vi "WFDC Compute Z Calibration.vi"(0 "Scan Positions File Name":string="Scan Positions.xml", 1 "User Close?":bool=TRUE, 2 "Half Shift":i32=7, 7 "Data Path":path, 11 "Error":errorcluster) -> (4 "Fit Slope":dbl=0.02 format="%#_6f", 8 "Fit Intercept":dbl=0.02, 13 "Ref Images":T1[](array[typedef]), 15 "Error":errorcluster)   [LabVIEW 2020]
uses:
  <vilib>/vision/Image Controls.llb/IMAQ Image.ctl
  WFDC Controls/WFDC Reference Image Info.ctl
  <vilib>/Utility/miscctls.llb/LVPointTypeDef.ctl
  <vilib>/Analysis/6fits.llb/Curve Fitting Criteria.ctl
  WFDC DLL and Testing/Visual Studio NCC Max Shift DLL/x64/Release/VSmaxShiftNCC.dll
  <vilib>/Analysis/NI_AALPro.lvlib
panel:
  out "Z Calibration":cluster{dbl[], dbl[]}[](graph)
  in  "Done":bool
  out "Wait Bar":i32(slide) scale=0.0..11.0
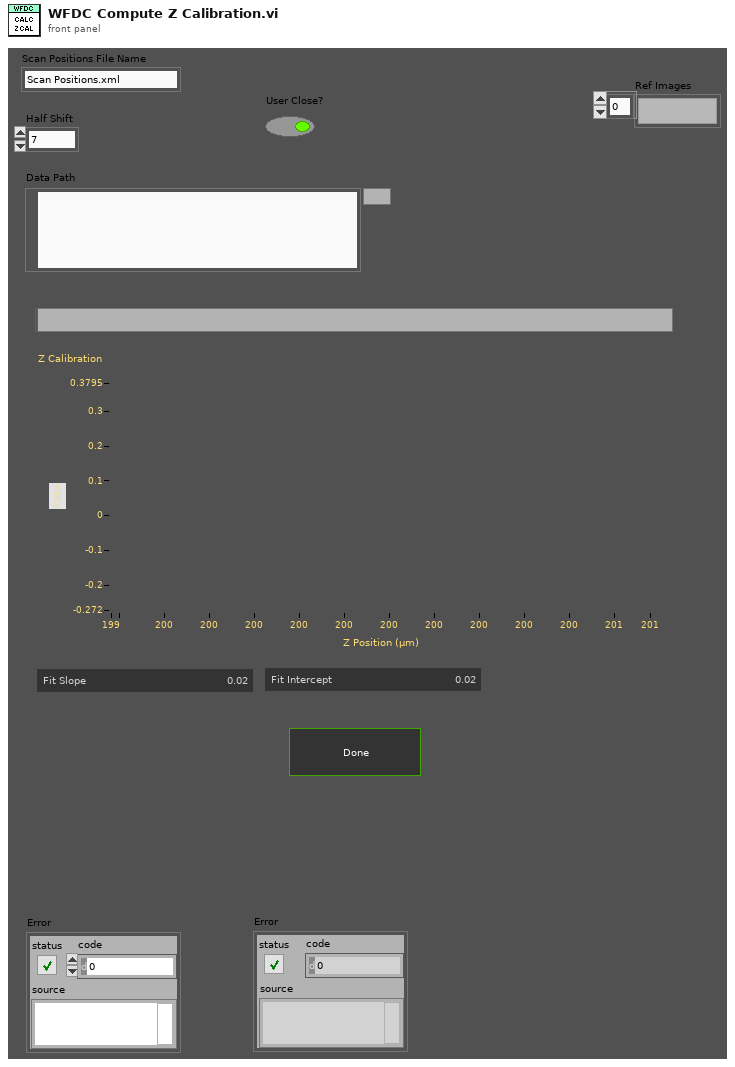
[diagram p1: front panel]
types:
  T1 = typedef "IMAQ Image.ctl" = refnum<image>
  T2 = enum16{"Always On", "Always Off", "Off While Running"}
  T3 = typedef "LVPointTypeDef.ctl" = cluster{"Horizontal":i16, "Vertical":i16}
  T4 = typedef "WFDC Reference Image Info.ctl" = cluster{"Image Path":path, "Z Position":dbl, "Number of Frames":u32}
  T5 = typedef "LVRectTypeDef.ctl" = cluster{"Left":i16, "Top":i16, "Right":i16, "Bottom":i16}
  T6 = typedef "LVBoundsTypeDef.ctl" = cluster{"Width":u32, "Height":u32}
  T7 = typedef "NI_AALPro.lvlib/Curve Fitting Criteria.ctl" = u16
  T8 = typedef "TIF Read Image Information.ctl" = cluster{"Byte Order":enum16{"big-endian, network order", "native, host order", "little-endian"}, "Width (pixels)":i32, "Height (pixels)":i32, "Bits per Pixel":u8, "Total Frames":u32, "First Frame Offset (bytes)":u32, "Frame Size (bytes)":u32}
  T9 = typedef "Image Type" = u32
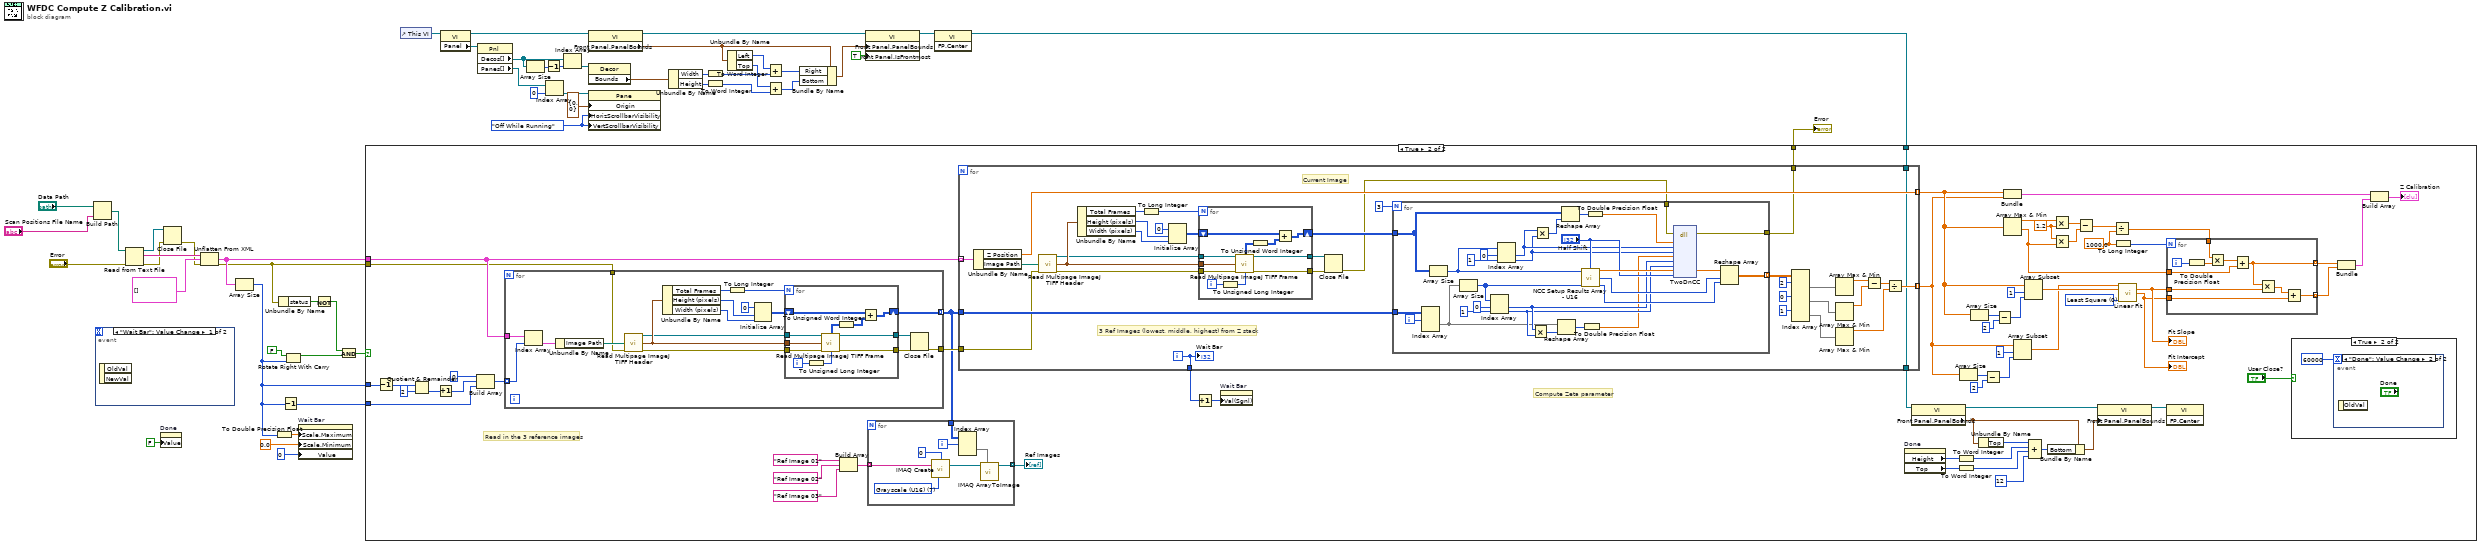
[diagram p0: block diagram]
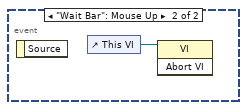
[diagram p2: hidden frame]
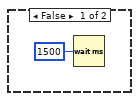
[diagram p4: hidden frame]
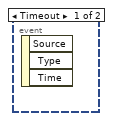
[diagram p5: hidden frame]
diagram:
  w25 = T2."Off While Running" ("Vertical Scrollbar Visibility")
  n1 = Build Path(base path="Data Path", name or relative path="Scan Positions File Name") -> (appended path=w1:path)
  n2 = event shown="[0] \"Wait Bar\": Value Change" {
    selector: _ -> [_ _]
    dyn-events: _ -> [_ _]
    timeout: _ -> [_ _]
    event "Wait Bar": Value Change {
      n3 = event-data() -> ()  [unwired: 1 in, 2 out]
    }
    event "Wait Bar": Mouse Up {
      n4 = event-data() -> ()  [unwired: 1 in, 1 out]
      n5 = control-ref of="This VI"() -> (w51:refnum<vi>)
      n6 = invoke class="VI" method="Abort VI"(reference=w51) -> ()  [unwired: 2 in, 3 out]
    }
  }
  n7 = Read from Text File(file (use dialog)=w1, error in="Error") -> (refnum out=w49:refnum<file>, text=w50:string, error out=w44:errorcluster)  [unwired: 2 in, 1 out]
  n8 = property on="Done" class="Bool (strict)"("Value"=FALSE ("Done")) -> ()  [unwired: 2 in, 2 out]
  n9 = Close File(refnum=w49, error in=w44) -> (error out=w43:errorcluster)  [unwired: 1 out]
  n10 = Unflatten From XML(xml string=w50, type=T4[] [], error in (no error)=w43) -> (value=w46:T4[], error out=w42:errorcluster)
  n11 = Array Size(array=w46) -> (size(s)=w9:i32)
  n12 = To Double Precision Float(number=w9) -> (double precision float=w8:dbl)
  n13 = Unbundle By Name(w42) -> ("status"=w41:bool)
  n14 = Decrement(x=w9) -> (x-1=w45:i32)
  n15 = Rotate Right With Carry(2:w9, 3:FALSE ("carry")) -> (1:w39:bool)  [unwired: 1 out]
  n16 = property on="Wait Bar" class="Slide (strict)"("Scale.Maximum"=w8, "Scale.Minimum"=0.0 ("Scale.Range:Minimum"), "Value"=0 ("Wait Bar")) -> ()  [unwired: 2 in, 2 out]
  n17 = Not(x=w41) -> (.not. x?=w40:bool)
  n18 = And(x=w40, y=w39) -> (x .and. y?=w38:bool)
  n19 = control-ref of="This VI"() -> (w12:refnum<vi>)
  n20 = property class="VI"(reference=w12) -> (reference out=w26:refnum<vi>, "Panel"=w19:refnum<vi>)  [unwired: 1 in, 1 out]
  n21 = property class="Pnl"(reference=w19) -> ("Decos[]"=w18:refnum<vi>[], "Panes[]"=w22:refnum<vi>[])  [unwired: 1 in, 2 out]
  n22 = Array Size(array=w18) -> (size(s)=w16:i32)
  n23 = Decrement(x=w16) -> (x-1=w17:i32)
  n24 = Index Array(array=w22, index=0) -> (element=w21:refnum<vi>)
  n25 = Index Array(array=w18, index=w17) -> (element=w24:refnum<vi>)
  n26 = property class="VI"(reference=w26) -> (reference out=w28:refnum<vi>, "Front Panel.PanelBounds"=w29:T5)  [unwired: 1 in, 1 out]
  n27 = property class="Decor"(reference=w24) -> ("Bounds"=w27:T6)  [unwired: 1 in, 2 out]
  n28 = property class="Pane"(reference=w21, "Origin"=T3 {"Horizontal"=0, "Vertical"=0}, "HorizScrollbarVisibility"=w25, "VertScrollbarVisibility"=w25) -> ()  [unwired: 1 in, 2 out]
  n29 = Unbundle By Name(w27) -> ("Width"=w32:u32, "Height"=w35:u32)
  n30 = To Word Integer(number=w32) -> (16bit integer=w34:i16)
  n31 = To Word Integer(number=w35) -> (16bit integer=w13:i16)
  n32 = Unbundle By Name(w29) -> ("Left"=w31:i16, "Top"=w15:i16)
  n33 = Add(x=w31, y=w34) -> (x+y=w33:i16)
  n34 = Add(x=w15, y=w13) -> (x+y=w14:i16)
  n35 = Bundle By Name(cluster=w29, "Right"=w33, "Bottom"=w14) -> (w30:T5)
  n36 = property class="VI"(reference=w28, "Front Panel.PanelBounds"=w30, "Front Panel.IsFrontmost"=TRUE ("Front Panel Window:Is Frontmost")) -> (reference out=w5:refnum<vi>)  [unwired: 1 in, 1 out]
  n37 = invoke class="VI" method="FP.Center"(reference=w5) -> (reference out=w4:refnum<vi>)  [unwired: 2 in, 2 out]
  n38 = case shown="True" w38 {
    tunnel: w9 -> [_ w115]
    tunnel: w46 -> [_ w107]
    tunnel: w45 -> [_ w109]
    tunnel: w42 -> [w52 w80]
    tunnel: [w52 w78] -> w36
    tunnel: w4 -> [_ w73]
    frame False {
    }
    frame True {
      w100 = 1000.0 ("y")
      w104 = 1.2 ("y")
      w106 = T7 0 items=["Least Square", "Least Absolute Residual", "Bisquare"] ("method")
      # "Compute Zeta parameter"
      # "Read in the 3 reference images"
      n39 = Decrement(x=w115) -> (x-1=w114:i32)
      n40 = Quotient & Remainder(x=w114, y=2) -> (floor(x/y)=w112:i32)  [unwired: 1 out]
      n41 = Increment(x=w112) -> (x+1=w111:i32)
      n42 = Build Array(0 ("element"), w111, w109) -> (w108:i32[])
      n43 = for {
        tunnel: w108 -> [w225] mode=indexing
        tunnel: w107 -> [w226]
        tunnel: [w212] -> w59 mode=indexing
        tunnel: [w210] -> w79
        tunnel: w80 -> [w209]
        n44 = Index Array(array=w226, index=w225) -> (element=w224:T4)
        n45 = Unbundle By Name(w224) -> ("Image Path"=w213:path)
        n46 = call "Read Multipage ImageJ TIFF Header.vi"("TIFF Path"=w213, "Error"=w209) -> ("TIF Ref"=w215:refnum<file>, "Image Info"=w217:T8, "Error"=w216:errorcluster)  [unwired: 11 in]
        n47 = Unbundle By Name(w217) -> ("Total Frames"=w218:u32, "Height (pixels)"=w222:i32, "Width (pixels)"=w221:i32)
        n48 = To Long Integer(number=w218) -> (32bit integer=w219:i32)
        n49 = Initialize Array(u16 0 ("element"), w222, w221) -> (w220:u16[][])
        n50 = for {
          N: w219 -> [_]
          tunnel: w215 -> [w237]
          tunnel: w217 -> [w236]
          tunnel: w216 -> [w235]
          shift-right: [w231] -> w212
          shift-left: w220 -> [w232]
          tunnel: [w230] -> w223
          tunnel: [w229] -> w211
          i -> [w234]
          n51 = To Unsigned Long Integer(number=w234) -> (unsigned 32bit integer=w233:u32)
          n52 = call "Read Multipage ImageJ TIFF Frame.vi"("TIF Ref"=w237, "Image Info"=w236, "Error"=w235, "Frame"=w233) -> ("U8 Image"=w228:u8[][], "TIF Ref (Dup)"=w230:refnum<file>, "Error"=w229:errorcluster)  [unwired: 8 in, 1 out]
          n53 = To Unsigned Word Integer(number=w228) -> (unsigned 16bit integer=w227:u16[][])
          n54 = Add(x=w232, y=w227) -> (x+y=w231:u16[][])
        }
        n55 = Close File(refnum=w223, error in=w211) -> (error out=w210:errorcluster)  [unwired: 1 out]
      }
      n56 = Build Array("Ref Image 01" ("Image Name"), "Ref Image 02" ("Image Name"), "Ref Image 03" ("Image Name")) -> (w63:string[])
      n57 = for {
        tunnel: w63 -> [w123] mode=indexing
        tunnel: w59 -> [w121]
        tunnel: [w118] -> w58 mode=indexing
        i -> [w119]
        w124 = T9 7 items=["Grayscale (U8)", "Grayscale (I16)", "Grayscale (SGL)", "Complex (CSG)", "RGB (U32)", "HSL (U32)", "RGB (U64)", "Grayscale (U16)"] ("Image Type")
        n58 = call "IMAQ Create"("Border Size"=0, "Image Name"=w123, "Image Type"=w124) -> ("New Image"=w122:T1)  [unwired: 2 in, 1 out]
        n59 = Index Array(array=w121, index (dim 0)=w119) -> (element=w120:u16[][])  [unwired: 2 in]
        n60 = call "IMAQ ArrayToImage"("Image Pixels (U16)"=w120, "Image"=w122) -> ("Image Out"=w118:T1)  [unwired: 8 in, 1 out]
      }
      "Ref Images" <- w58
      n61 = for {
        tunnel: w59 -> [w169]
        tunnel: w107 -> [w168] mode=indexing
        tunnel: [w167] -> w82 mode=indexing
        tunnel: [w166] -> w81 mode=indexing
        tunnel: w79 -> [w165]
        tunnel: [w164] -> w78
        tunnel: [w163] -> w77
        tunnel: w73 -> [w162]
        tunnel: [w162] -> w72
        i -> [w163]
        # "Current Image"
        # "3 Ref Images (lowest, middle, highest) from Z stack"
        n62 = Unbundle By Name(w168) -> ("Z Position"=w167:dbl, "Image Path"=w151:path)
        n63 = call "Read Multipage ImageJ TIFF Header.vi"("TIFF Path"=w151, "Error"=w165) -> ("TIF Ref"=w153:refnum<file>, "Image Info"=w155:T8, "Error"=w154:errorcluster)  [unwired: 11 in]
        n64 = Unbundle By Name(w155) -> ("Total Frames"=w156:u32, "Height (pixels)"=w160:i32, "Width (pixels)"=w159:i32)
        n65 = To Long Integer(number=w156) -> (32bit integer=w157:i32)
        n66 = Initialize Array(u16 0 ("element"), w160, w159) -> (w158:u16[][])
        n67 = for {
          N: w157 -> [_]
          tunnel: w153 -> [w208]
          tunnel: w155 -> [w207]
          tunnel: w154 -> [w206]
          shift-right: [w202] -> w149
          shift-left: w158 -> [w203]
          tunnel: [w201] -> w161
          tunnel: [w200] -> w137
          i -> [w205]
          n68 = To Unsigned Long Integer(number=w205) -> (unsigned 32bit integer=w204:u32)
          n69 = call "Read Multipage ImageJ TIFF Frame.vi"("TIF Ref"=w208, "Image Info"=w207, "Error"=w206, "Frame"=w204) -> ("U8 Image"=w199:u8[][], "TIF Ref (Dup)"=w201:refnum<file>, "Error"=w200:errorcluster)  [unwired: 8 in, 1 out]
          n70 = To Unsigned Word Integer(number=w199) -> (unsigned 16bit integer=w198:u16[][])
          n71 = Add(x=w203, y=w198) -> (x+y=w202:u16[][])
        }
        n72 = Close File(refnum=w161, error in=w137) -> (error out=w136:errorcluster)  [unwired: 1 out]
        n73 = for {
          N: 3 -> [_]
          tunnel: w169 -> [w197]
          tunnel: w149 -> [w177]
          tunnel: [w172] -> w148 mode=indexing
          tunnel: w136 -> [w171]
          tunnel: [w170] -> w164
          i -> [w196]
          n74 = Index Array(array=w197, index (dim 0)=w196) -> (element=w184:u16[][])  [unwired: 2 in]
          n75 = Array Size(array=w177) -> (size(s)=w179:i32[])
          n76 = Array Size(array=w184) -> (size(s)=w190:i32[])
          n77 = Index Array(array=w190, index #1=0 ("index"), index #2=1 ("index")) -> (element #1=w187:i32, element #2=w186:i32)
          n78 = Index Array(array=w179, index #1=0 ("index"), index #2=1 ("index")) -> (element #1=w175:i32, element #2=w174:i32)
          n79 = Multiply(x=w187, y=w186) -> (x*y=w185:i32)
          n80 = Multiply(x=w175, y=w174) -> (x*y=w173:i32)
          n81 = Reshape Array(w184, w185) -> (w183:u16[])
          n82 = Reshape Array(w177, w173) -> (w178:u16[])
          n83 = call "NCC Setup Results Array - U16.vi"("Image 01 Size"=w179, "Half Shift"="Half Shift", "Image 02 Size"=w190) -> ("NCC Results Array"=w195:dbl[], "Result Rows"=w192:i32, "Result Columns"=w193:i32)  [unwired: 10 in]
          n84 = To Double Precision Float(number=w183) -> (double precision float=w182:dbl[])
          n85 = To Double Precision Float(number=w178) -> (double precision float=w176:dbl[])
          n86 = dll-call lib="C:/Users/George Sirinakis/Documents/Microscope-Control/Microscope Modules/Wide Field Drift Correction/WFDC DLL and Testing/Visual Studio NCC Max Shift DLL/x64/Release/VSmaxShiftNCC.dll" fn="TwoDnCC"(error in=w171, "im01"=w176, "im01rowSize"=w175, "im01colSize"=w174, "im02"=w182, "im02rowSize"=w187, "im02ColSize"=w186, "theResult"=w195, "halfShift"="Half Shift") -> (error out=w170:errorcluster, "theResult"=w194:dbl[])  [unwired: 10 in, 1 out]
          n87 = Reshape Array(w194, w192, w193) -> (w172:dbl[][])
        }
        n88 = Index Array(array=w148, index (dim 0) #1=2 ("index (page)"), index (dim 0) #2=0 ("index (page)"), index (dim 0) #3=1 ("index (page)")) -> (element #1=w140:dbl[][], element #2=w138:dbl[][], element #3=w139:dbl[][])  [unwired: 6 in]
        n89 = Array Max & Min(array=w140) -> (max value=w144:dbl)  [unwired: 3 out]
        n90 = Array Max & Min(array=w138) -> (max value=w143:dbl)  [unwired: 3 out]
        n91 = Array Max & Min(array=w139) -> (max value=w141:dbl)  [unwired: 3 out]
        n92 = Subtract(x=w144, y=w143) -> (x-y=w142:dbl)
        n93 = Divide(x=w142, y=w141) -> (x/y=w166:dbl)
        "Wait Bar" <- w163
      }
      n94 = Increment(x=w77) -> (x+1=w76:i32)
      n95 = property on="Wait Bar" class="Slide (strict)"("Val(Sgnl)"=w76) -> ()  [unwired: 2 in, 2 out]
      n96 = property on="Done" class="Bool (strict)"() -> ("Height"=w68:u32, "Top"=w67:i32)  [unwired: 2 in, 2 out]
      n97 = property class="VI"(reference=w72) -> (reference out=w74:refnum<vi>, "Front Panel.PanelBounds"=w71:T5)  [unwired: 1 in, 1 out]
      n98 = To Word Integer(number=w68) -> (16bit integer=w66:i16)
      n99 = To Word Integer(number=w67) -> (16bit integer=w65:i16)
      n100 = Array Size(array=w81) -> (size(s)=w91:i32)
      n101 = Array Size(array=w82) -> (size(s)=w88:i32)
      n102 = Unbundle By Name(w71) -> ("Top"=w70:i16)
      n103 = Subtract(x=w91, y=2) -> (x-y=w89:i32)
      n104 = Subtract(x=w88, y=2) -> (x-y=w87:i32)
      n105 = Bundle(w82, w81) -> (w94:cluster{dbl[], dbl[]})  [unwired: 1 in]
      n106 = Array Max & Min(array=w82) -> (max value=w105:dbl, min value=w98:dbl)  [unwired: 2 out]
      n107 = Array Subset(array=w81, index=1, length=w89) -> (w83:dbl[])
      n108 = Array Subset(array=w82, index=1, length=w87) -> (w84:dbl[])
      n109 = Compound Arithmetic op=ADD(w70, w66, w65, i16 12) -> (w69:i16)
      n110 = Bundle By Name(cluster=w71, "Bottom"=w69) -> (w75:T5)
      n111 = Multiply(x=w105, y=w104) -> (x*y=w103:dbl)
      n112 = Multiply(x=w104, y=w98) -> (x*y=w102:dbl)
      n113 = Subtract(x=w103, y=w102) -> (x-y=w101:dbl)
      n114 = property class="VI"(reference=w74, "Front Panel.PanelBounds"=w75) -> (reference out=w57:refnum<vi>)  [unwired: 1 in, 1 out]
      n115 = Divide(x=w101, y=w100) -> (x/y=w97:dbl)
      n116 = To Long Integer(number=w100) -> (32bit integer=w99:i32)
      n117 = call <vilib>:"Linear Fit.vi"("Y"=w83, "X"=w84, "method"=w106) -> ("slope"=w56:dbl, "intercept"=w55:dbl)  [unwired: 8 in, 3 out]
      "Fit Slope" <- w56
      "Fit Intercept" <- w55
      n118 = for {
        N: w99 -> [_]
        tunnel: w98 -> [w131]
        tunnel: w97 -> [w133]
        tunnel: [w130] -> w96 mode=indexing
        tunnel: w55 -> [w127]
        tunnel: w56 -> [w129]
        tunnel: [w126] -> w95 mode=indexing
        i -> [w135]
        n119 = To Double Precision Float(number=w135) -> (double precision float=w134:dbl)
        n120 = Multiply(x=w133, y=w134) -> (x*y=w132:dbl)
        n121 = Add(x=w132, y=w131) -> (x+y=w130:dbl)
        n122 = Multiply(x=w130, y=w129) -> (x*y=w128:dbl)
        n123 = Add(x=w128, y=w127) -> (x+y=w126:dbl)
      }
      n124 = invoke class="VI" method="FP.Center"(reference=w57) -> ()  [unwired: 2 in, 3 out]
      n125 = case shown="True" "User Close?" {
        frame False {
          n126 = Wait (ms)(milliseconds to wait=u32 1500) -> ()  [unwired: 1 out]
        }
        frame True {
          n127 = event shown="[1] \"Done\": Value Change" {
            selector: _ -> [_ _]
            dyn-events: _ -> [_ _]
            timeout: 60000 -> [_ _]
            event Timeout {
              n128 = event-data() -> ()  [unwired: 1 in, 3 out]
            }
            event "Done": Value Change {
              n129 = event-data() -> ()  [unwired: 1 in, 1 out]
            }
          }
        }
      }
      n130 = Bundle(w96, w95) -> (w93:cluster{dbl[], dbl[]})  [unwired: 1 in]
      n131 = Build Array(w94, w93) -> (→"Z Calibration":cluster{dbl[], dbl[]}[])
    }
  }
  "Error" <- w36
